vi "基础价格.vi"(8 "error in (no error)":errorcluster caption="错误输入（无错误）", 11 "招牌奶茶 输入":refnum<class "招牌奶茶.lvclass">) -> (0 "error out":errorcluster caption="错误输出", 2 "基础价格":dbl, 3 "招牌奶茶 输出":refnum<class "招牌奶茶.lvclass">)   [LabVIEW 2016, in "招牌奶茶.lvclass"]
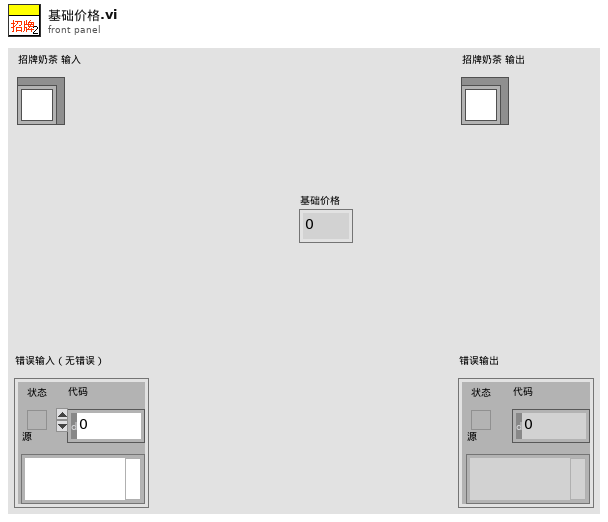
[diagram p1: front panel]
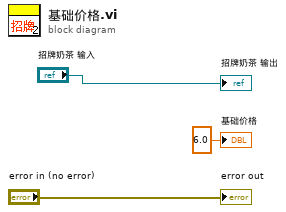
[diagram p0: block diagram]
diagram:
  "error out" <- "error in (no error)"
  "招牌奶茶 输出" <- "招牌奶茶 输入"
  "基础价格" <- 6.0 ("基础价格")
